vi "Magnet Set Remote.vi"   [LabVIEW 2009, in "Magnet.lvclass"]
uses:
  Magnet.lvclass
  Global/Power Supply.vi
  Global/Temp Controller.vi
  Global/Level Meter.vi
types:
  T1 = typedef "OxfordAddress.ctl" = cluster{"Com Port":i32, "ISOBUS Address":i32, "GPIB Address":i16, "Communication":enum16{"RS232", "ISOBUS", "GPIB", "Gateway"}}
  T2 = cluster{"Address":T1, "ILM Name":string, "Display Channel":i32[]}
  T3 = typedef "ITCIO.ctl" = cluster{"Address":T1, "Version":T4, "Ch 1 dec places":i16, "Ch 2 dec places":i16, "Ch 3 dec places":i16, "Ch1 Name":string, "Ch2 Name":string, "Ch3 Name":string}
  T4 = typedef "ITCVersion.ctl" = enum16{"ITC502", "ITC503", "ITC601"}
  T5 = typedef "PSIO.ctl" = cluster{"Address":T1, "Version":enum16{"PS", "IPS"}}
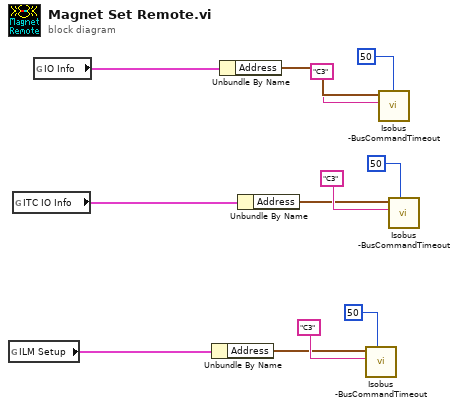
[diagram p0: block diagram]
diagram:
  n1 = global read "Level Meter.vi" "ILM Setup"() -> (w1:T2)
  n2 = global read "Temp Controller.vi" "ITC IO Info"() -> (w2:T3)
  n3 = global read "Power Supply.vi" "IO Info"() -> (w3:T5)
  n4 = Unbundle By Name(w1) -> ("Address"=w5:T1)
  n5 = Unbundle By Name(w3) -> ("Address"=w12:T1)
  n6 = Unbundle By Name(w2) -> ("Address"=w8:T1)
  n7 = call "Isobus -BusCommandTimeout.vi"("Timeout (ms)"=50, "Command"="C3", "Address"=w5) -> ()  [unwired: 6 out]
  n8 = call "Isobus -BusCommandTimeout.vi"("Timeout (ms)"=50, "Command"="C3", "Address"=w12) -> ()  [unwired: 6 out]
  n9 = call "Isobus -BusCommandTimeout.vi"("Timeout (ms)"=50, "Command"="C3", "Address"=w8) -> ()  [unwired: 6 out]
